vi "Remove UIP.vi"(8 "Error In":errorcluster, 10 "UIP":refnum<class "UIP Interface.lvclass">, 11 "UIM In":refnum<data-value>) -> (0 "Error Out":errorcluster, 3 "UIM Out":refnum<data-value>)   [LabVIEW 2020, in "UIM.lvlib" / "UIM.lvclass"]
doc: "Remove a UIP from the UIM by path. If no UIP with provided path is found, nothing happens."
uses:
  UIM.lvclass
  UIP Interface/UIP Interface.lvclass
  UIM.lvclass/UIM.ctl
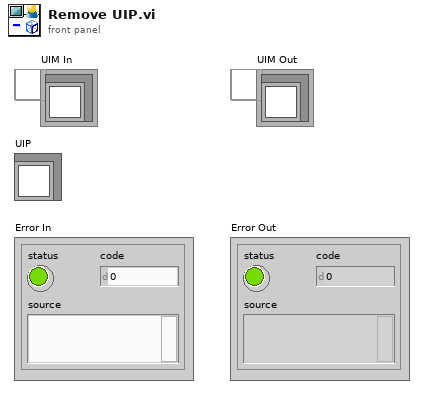
[diagram p1: front panel]
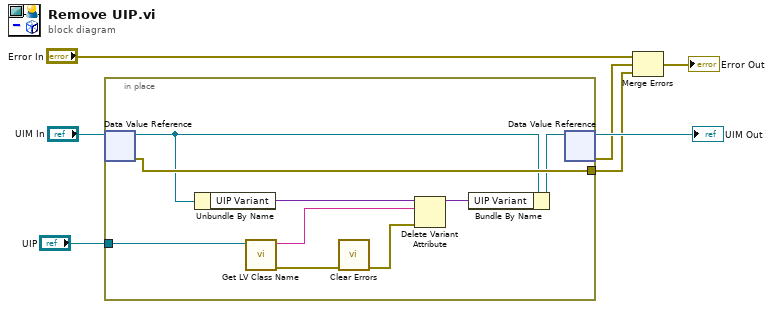
[diagram p0: block diagram]
diagram:
  n1 = in-place {
    in-place-border: [w16] -> w3
    in-place-border: "UIP" -> [w8]
    n2 = in-place-dvr #1("UIM In") -> (w15:refnum<class "UIM.lvclass">, w16:errorcluster)
    n3 = Unbundle By Name(w15) -> ("UIP Variant"=w13:variant)
    n4 = call <vilib>:"Get LV Class Name.vi"("object"=w8) -> ("error out"=w14:errorcluster, "class name"=w12:string)  [unwired: 9 in]
    n5 = call <vilib>:"Clear Errors.vi"("error in (no error)"=w14) -> ("error out"=w11:errorcluster)  [unwired: 5 in, 1 out]
    n6 = Delete Variant Attribute(4:w11, 6:w12, 7:w13) -> (3:w9:variant)  [unwired: 2 out]
    n7 = Bundle By Name(cluster=w15, "UIP Variant"=w9) -> (w10:refnum<class "UIM.lvclass">)
    n8 = in-place-dvr #1(w10) -> (→"UIM Out":refnum<data-value>, w2:errorcluster)
  }
  n9 = Merge Errors("Error In", w2, w3) -> (→"Error Out":errorcluster)
